vi "Configure Refreshing.vi"(8 "error in (no error)":errorcluster, 10 "Refresh?":bool, 11 "Debugger In":refnum<class "Debugger.lvclass">) -> (0 "error out":errorcluster, 3 "Debugger Out":refnum<class "Debugger.lvclass">)   [LabVIEW 2020, in "Debugger.lvclass"]
uses:
  Debugger.lvclass
  C:/Git/astemes-triarc-debugger/source/Process/Debug Process.lvclass
  Process/Debug Process.lvclass/Debug Process.ctl
  Debugger.lvclass/Debugger.ctl
  <vilib>/Utility/error.llb/Clear Errors.vi
  <vilib>/Utility/error.llb/Error Cluster From Error Code.vi
  Process/Debug Process.lvclass
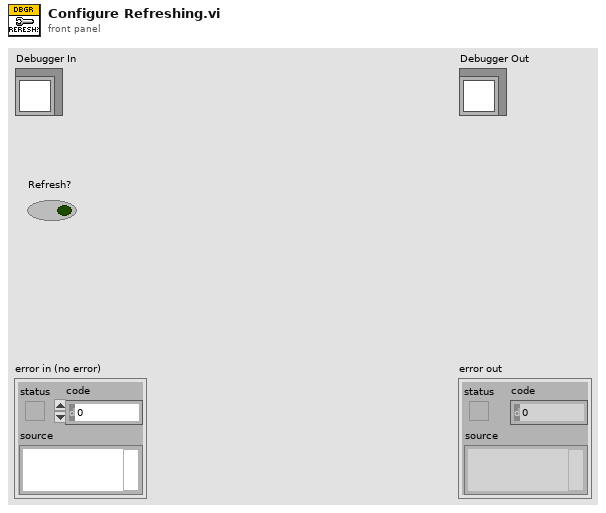
[diagram p1: front panel]
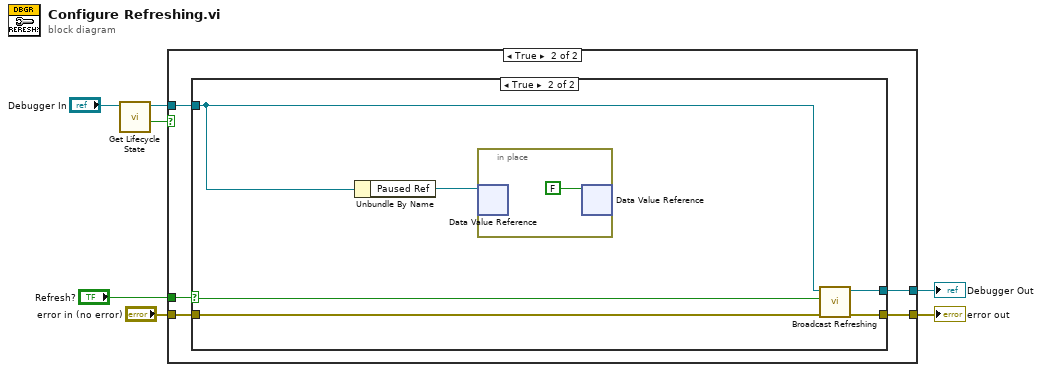
[diagram p0: block diagram]
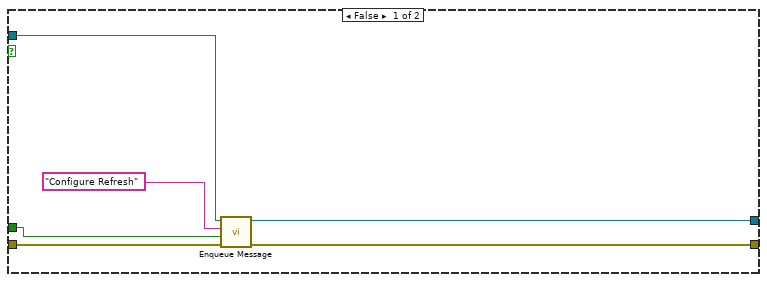
[diagram p2: hidden frame]
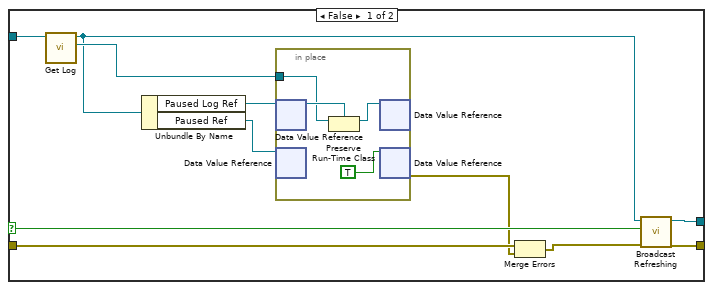
[diagram p3: hidden frame]
diagram:
  n1 = call "Get Lifecycle State.vi"("Process In"="Debugger In") -> ("In Process Loop?"=w2:bool, "Process Out"=w3:refnum<class "Debugger.lvclass">)  [unwired: 7 in, 2 out]
  n2 = case shown="True" w2 {
    tunnel: "error in (no error)" -> [w13 w18]
    tunnel: [w12 w17] -> w6
    tunnel: [w11 w16] -> w4
    tunnel: w3 -> [w9 w14]
    tunnel: "Refresh?" -> [w8 w15]
    frame False {
      n3 = call "Enqueue Message.vi"("error in (no error)"=w13, "Message Data"=w8, "Message"="Configure Refresh", "Process In"=w9) -> ("error out"=w12:errorcluster, "Process Out"=w11:refnum<class "Debugger.lvclass">)  [unwired: 6 in]
    }
    frame True {
      n4 = case shown="True" w15 {
        selector: w15 -> [w27 w36]
        tunnel: w18 -> [w20 w37]
        tunnel: [w29 w38] -> w17
        tunnel: [w28 w39] -> w16
        tunnel: w14 -> [w25 w34]
        frame False {
          n5 = call "Get Log.vi"("Debugger in"=w25) -> ("Log"=w26:refnum<class "Debug Log.lvclass">, "Debugger out"=w24:refnum<class "Debugger.lvclass">)  [unwired: 8 in, 1 out]
          n6 = Unbundle By Name(w24) -> ("Paused Log Ref"=w23:refnum<data-value>, "Paused Ref"=w22:refnum<data-value>)
          n7 = in-place {
            in-place-border: w26 -> [w31]
            n8 = in-place-dvr #1(w23) -> (w32:refnum<class "Debug Log.lvclass">)  [unwired: 1 out]
            n9 = in-place-dvr #2(w22) -> ()  [unwired: 2 out]
            n10 = Preserve Run-Time Class(object in=w31, 2:w32) -> (object out=w33:refnum<class "Debug Log.lvclass">)  [unwired: 1 in, 1 out]
            n11 = in-place-dvr #1(w33) -> ()  [unwired: 2 out]
            n12 = in-place-dvr #2(TRUE ("data value")) -> (w19:errorcluster)  [unwired: 1 out]
          }
          n13 = Merge Errors(w20, w19) -> (w21:errorcluster)
          n14 = call "Broadcast Refreshing.vi"("error in (no error)"=w21, "Refresh?"=w27, "Debugger in"=w24) -> ("error out"=w29:errorcluster, "Debugger out"=w28:refnum<class "Debugger.lvclass">)  [unwired: 7 in]
        }
        frame True {
          n15 = Unbundle By Name(w34) -> ("Paused Ref"=w35:refnum<data-value>)
          n16 = in-place {
            n17 = in-place-dvr #3(w35) -> ()  [unwired: 2 out]
            n18 = in-place-dvr #3(FALSE ("data value")) -> ()  [unwired: 2 out]
          }
          n19 = call "Broadcast Refreshing.vi"("error in (no error)"=w37, "Refresh?"=w36, "Debugger in"=w34) -> ("error out"=w38:errorcluster, "Debugger out"=w39:refnum<class "Debugger.lvclass">)  [unwired: 7 in]
        }
      }
    }
  }
  "error out" <- w6
  "Debugger Out" <- w4
